vi "ENCODERS AUTO SUBVI.vi"   [LabVIEW 2011]
uses:
  Robot Global Data.vi
types:
  T1 = typedef "WPI_RobotDriveDevRef.ctl" = cluster{"DevStatus":errorcluster, "Motors[]":T2[], "Square Inputs":bool, "Max Output":dbl, "Isochronous":bool}
  T2 = typedef "WPI_MotorControlDeviceRef.ctl" = cluster{"DeviceStatus":errorcluster, "Type":enum16{"PWM", "CAN"}, "PWM":cluster{"Digital Module":T3, "PWM Channel":T4, "DeadBand":T5}, "CAN":cluster{"Device Number":u8, "Control Mode":T6, "Semaphore":T7, "Max Vout":dbl}, "Invert":bool, "TransformRef":T8, "InvTransformRef":T8}
  T3 = typedef "FPGA_TypedefDigitalModule.ctl" = enum16{"Digital Module 1", "Digital Module 2"}
  T4 = typedef "FPGA_DIOPWMChannel.ctl" = enum8{"PWM 1", "PWM 2", "PWM 3", "PWM 4", "PWM 5", "PWM 6", "PWM 7", "PWM 8", "PWM 9", "PWM 10", "Invalid"}
  T5 = typedef "WPI_PWMDeadband.ctl" = cluster{"Name":string, "maxPositivePwm":i32, "minPositivePwm":i32, "centerPwm":i32, "maxNegativePwm":i32, "minNegativePwm":i32, "angularRange":u16}
  T6 = typedef "WPI_CANJaguar_ControlMode.ctl" = enum8{"Percent VBus", "Current", "Speed", "Position", "Voltage"}
  T7 = typedef "Semaphore RefNum" = refnum<k1>
  T8 = typedef "WPI_PWMTransform_ConPane.ctl" = refnum<vi>
  T9 = typedef "WPI_DigitalInputDevRef.ctl" = cluster{"DevStatus":errorcluster, "DIO Channel":T10, "Digital Module":T3}
  T10 = typedef "FPGA_DIOChannel.ctl" = enum8{"DIO 1", "DIO 2", "DIO 3", "DIO 4", "DIO 5", "DIO 6", "DIO 7", "DIO 8", "DIO 9", "DIO 10", "DIO 11", "DIO 12", "DIO 13", "DIO 14", "Invalid"}
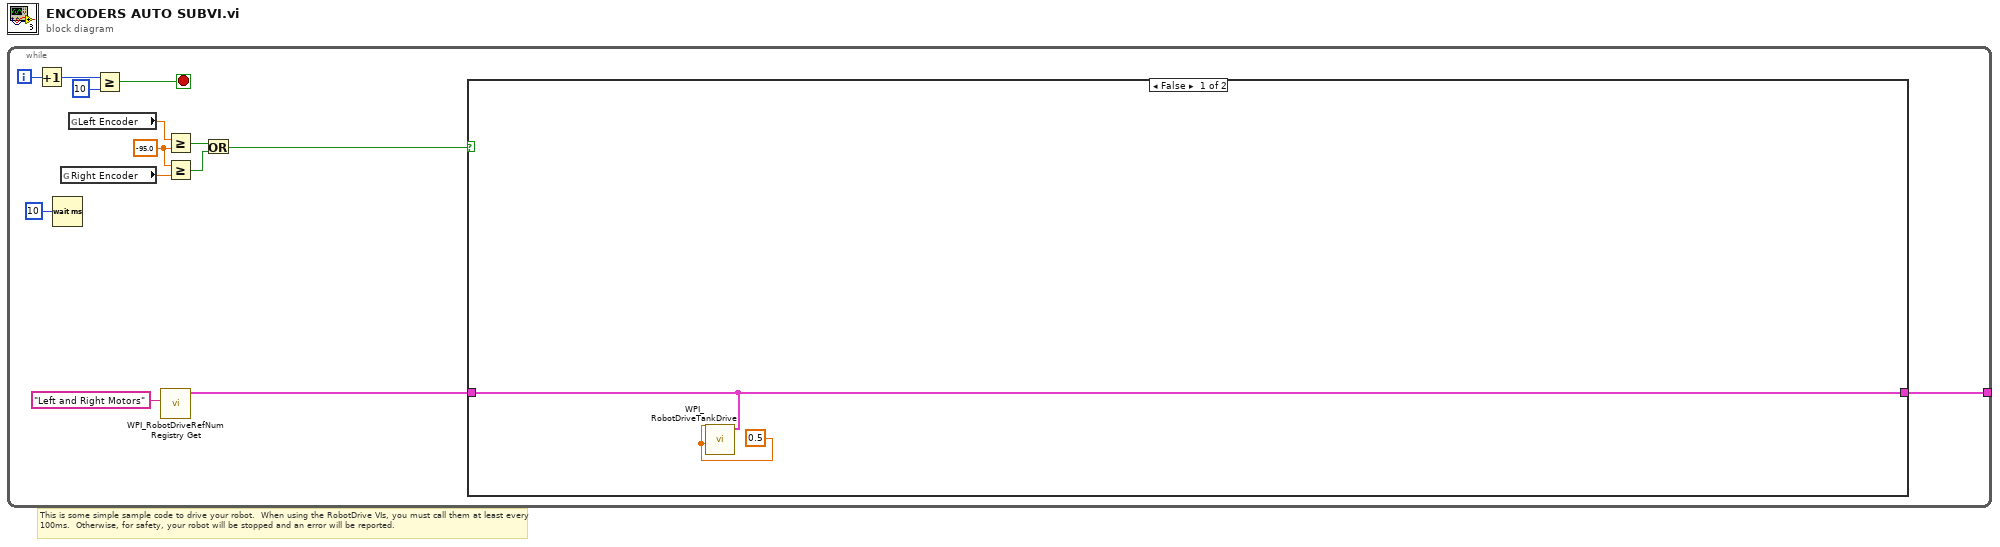
[diagram p0: block diagram]
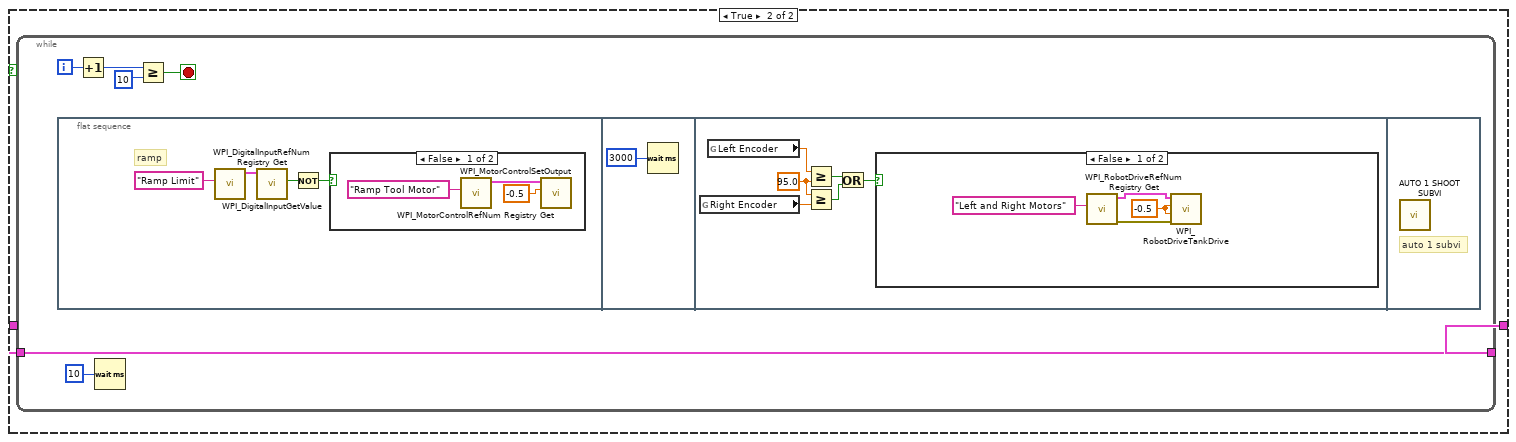
[diagram p2: hidden frame]
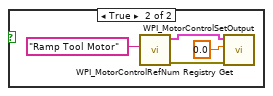
[diagram p3: hidden frame]
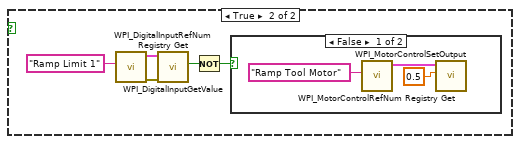
[diagram p4: hidden frame]
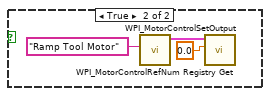
[diagram p5: hidden frame]
diagram:
  # "This is some simple sample code to drive your robot.  When using the RobotDrive VIs, you must call them at least every 100ms.  Otherwise, for safety, your robot will be stopped and an error will be reported."
  n1 = while {
    tunnel: [w1] -> _
    i -> [w8]
    stop <- w9 stop-if-true
    w4 = -95.0 ("y")
    n2 = Increment(x=w8) -> (x+1=w11:i32)
    n3 = Wait (ms)(milliseconds to wait=u32 10) -> ()  [unwired: 1 out]
    n4 = global read "Robot Global Data.vi" "Right Encoder"() -> (w5:dbl)
    n5 = global read "Robot Global Data.vi" "Left Encoder"() -> (w6:dbl)
    n6 = Greater Or Equal?(x=w11, y=10) -> (x >= y?=w9:bool)
    n7 = call <vilib>:"WPI_RobotDriveRefNum Registry Get.vi"("refnum name"="Left and Right Motors") -> ("RobotDriveDevRef"=w2:T1)  [unwired: 1 in, 9 out]
    n8 = Greater Or Equal?(x=w6, y=w4) -> (x >= y?=w14:bool)
    n9 = Greater Or Equal?(x=w4, y=w5) -> (x >= y?=w13:bool)
    n10 = Or(x=w14, y=w13) -> (x .or. y?=w12:bool)
    n11 = case shown="False" w12 {
      tunnel: w2 -> [w15 w18]
      tunnel: [w15 w17] -> w1
      frame False {
        w16 = 0.5 ("Left axis value")
        n12 = call <vilib>:"WPI_RobotDriveTankDrive.vi"("Right axis value"=w16, "Left axis value"=w16, "RobotDriveDevRef"=w15) -> ()  [unwired: 1 in, 8 out]
      }
      frame True {
        n13 = while {
          tunnel: [w20] -> w17
          tunnel: w18 -> [w20]
          i -> [w22]
          stop <- w21 stop-if-true
          n14 = flat-sequence {
            frame #0 {
              # "ramp"
              n15 = call <vilib>:"WPI_DigitalInputRefNum Registry Get.vi"("refnum name"="Ramp Limit") -> ("DigitalInputDevRef"=w27:T9)  [unwired: 9 in, 1 out]
              n16 = call <vilib>:"WPI_DigitalInputGetValue.vi"("DigitalInputDevRef"=w27) -> ("Value"=w26:bool)  [unwired: 8 in, 2 out]
              n17 = Not(x=w26) -> (.not. x?=w25:bool)
              n18 = case shown="False" w25 {
                frame False {
                  n19 = call <vilib>:"WPI_MotorControlRefNum Registry Get.vi"("refnum name"="Ramp Tool Motor") -> ("MotorControlDevRef"=w31:T2)  [unwired: 9 in, 1 out]
                  n20 = call <vilib>:"WPI_MotorControlSetOutput.vi"("Output"=-0.5, "MotorControlDevRef"=w31) -> ()  [unwired: 8 in, 2 out]
                }
                frame True {
                  n21 = call <vilib>:"WPI_MotorControlRefNum Registry Get.vi"("refnum name"="Ramp Tool Motor") -> ("error out"=w34:errorcluster, "MotorControlDevRef"=w35:T2)  [unwired: 9 in]
                  n22 = call <vilib>:"WPI_MotorControlSetOutput.vi"("error in (no error)"=w34, "Output"=0.0, "MotorControlDevRef"=w35) -> ()  [unwired: 7 in, 2 out]
                }
              }
            }
            frame #1 {
              n23 = Wait (ms)(milliseconds to wait=u32 3000) -> ()  [unwired: 1 out]
            }
            frame #2 {
              w38 = 95.0 ("y")
              n24 = global read "Robot Global Data.vi" "Right Encoder"() -> (w39:dbl)
              n25 = global read "Robot Global Data.vi" "Left Encoder"() -> (w40:dbl)
              n26 = Greater Or Equal?(x=w40, y=w38) -> (x >= y?=w42:bool)
              n27 = Greater Or Equal?(x=w38, y=w39) -> (x >= y?=w41:bool)
              n28 = Or(x=w42, y=w41) -> (x .or. y?=w37:bool)
              n29 = case shown="False" w37 {
                frame False {
                  w46 = -0.5 ("Left axis value")
                  n30 = call <vilib>:"WPI_RobotDriveRefNum Registry Get.vi"("refnum name"="Left and Right Motors") -> ("error out"=w44:errorcluster, "RobotDriveDevRef"=w45:T1)  [unwired: 1 in, 8 out]
                  n31 = call <vilib>:"WPI_RobotDriveTankDrive.vi"("error in (no error)"=w44, "Right axis value"=w46, "Left axis value"=w46, "RobotDriveDevRef"=w45) -> ()  [unwired: 8 out]
                }
                frame True {
                  n32 = call <vilib>:"WPI_DigitalInputRefNum Registry Get.vi"("refnum name"="Ramp Limit 1") -> ("error out"=w51:errorcluster, "DigitalInputDevRef"=w50:T9)  [unwired: 9 in]
                  n33 = call <vilib>:"WPI_DigitalInputGetValue.vi"("error in (no error)"=w51, "DigitalInputDevRef"=w50) -> ("Value"=w48:bool)  [unwired: 7 in, 2 out]
                  n34 = Not(x=w48) -> (.not. x?=w47:bool)
                  n35 = case shown="False" w47 {
                    frame False {
                      n36 = call <vilib>:"WPI_MotorControlRefNum Registry Get.vi"("refnum name"="Ramp Tool Motor") -> ("MotorControlDevRef"=w54:T2)  [unwired: 9 in, 1 out]
                      n37 = call <vilib>:"WPI_MotorControlSetOutput.vi"("Output"=0.5, "MotorControlDevRef"=w54) -> ()  [unwired: 8 in, 2 out]
                    }
                    frame True {
                      n38 = call <vilib>:"WPI_MotorControlRefNum Registry Get.vi"("refnum name"="Ramp Tool Motor") -> ("MotorControlDevRef"=w55:T2)  [unwired: 9 in, 1 out]
                      n39 = call <vilib>:"WPI_MotorControlSetOutput.vi"("Output"=0.0, "MotorControlDevRef"=w55) -> ()  [unwired: 8 in, 2 out]
                    }
                  }
                }
              }
            }
            frame #3 {
              # "auto 1 subvi"
              n40 = call "AUTO 1 SHOOT SUBVI.vi"() -> ()  [unwired: 12 in]
            }
          }
          n41 = Increment(x=w22) -> (x+1=w23:i32)
          n42 = Wait (ms)(milliseconds to wait=u32 10) -> ()  [unwired: 1 out]
          n43 = Greater Or Equal?(x=w23, y=10) -> (x >= y?=w21:bool)
        }
      }
    }
  }
